vi "Untitled 2 (SubVI).vi"(11 "Cluster":T1) -> (3 "appended array":u32[](array[numeric]))   [LabVIEW 2015, in "Igor.lvclass"]
uses:
  Igor.lvclass
  Memory.ctl
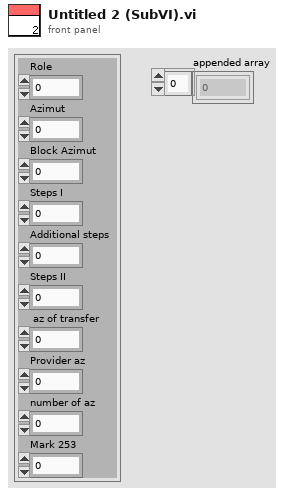
[diagram p1: front panel]
types:
  T1 = typedef "Memory.ctl" = cluster{"Role":i32, "Azimut":i32, "Block Azimut":i32, "Steps I":u32, "Additional steps":i32, "Steps II":u32, " az of transfer":u32, "Provider az":u32, "number of az":u32, "Mark 253":u32}
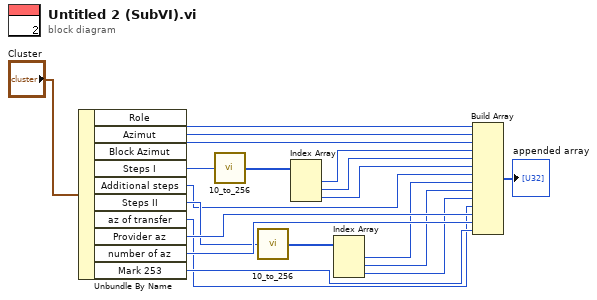
[diagram p0: block diagram]
diagram:
  n1 = Unbundle By Name("Cluster") -> ("Role"=w2:i32, "Azimut"=w3:i32, "Block Azimut"=w4:i32, "Steps I"=w6:u32, "Additional steps"=w10:i32, "Steps II"=w12:u32, "az of transfer"=w16:u32, "Provider az"=w17:u32, "number of az"=w18:u32, "Mark 253"=w19:u32)
  n2 = call "10_to_256.vi"("Decimal"=w6) -> ("256"=w5:u8[])
  n3 = call "10_to_256.vi"("Decimal"=w12) -> ("256"=w11:u8[])
  n4 = Index Array(array=w5) -> (element #1=w7:u8, element #2=w8:u8, element #3=w9:u8)  [unwired: 3 in]
  n5 = Index Array(array=w11) -> (element #1=w13:u8, element #2=w14:u8, element #3=w15:u8)  [unwired: 3 in]
  n6 = Build Array(w2, w3, w4, w7, w8, w9, w10, w13, w14, w15, w16, w17, w18, w19) -> (→"appended array":u32[])
